vi "Add PV Protocols to FGV.vi"(8 "Error In":errorcluster, 10 "PV Protocol Section":string="PV_Protocols", 11 "CS++Factory":refnum<class "CS++Factory.lvclass">) -> (0 "Error Out":errorcluster)   [LabVIEW 2014, in "CS++ProcessVariables.lvlib"]
doc: "Read PV Protocols from configuration data to FGV."
uses:
  CS++ProcessVariables.lvlib
  CS++BaseClasses/Factory/CS++Factory.lvclass
  PVConnection/PVConnection.lvclass
  Libraries/Base/FGV Action.ctl
  Libraries/Base/CS++Base.lvlib
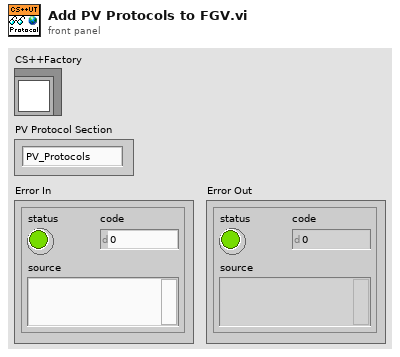
[diagram p1: front panel]
types:
  T1 = typedef "CS++Base.lvlib/FGV Action.ctl" = enum16{"add", "replace", "read", "remove", "reset", "get attributes"}
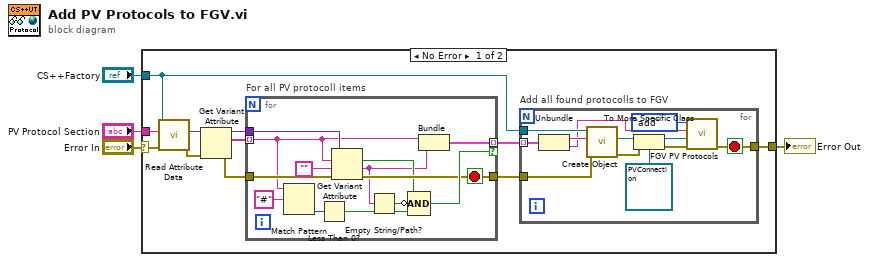
[diagram p0: block diagram]
diagram:
  n1 = case shown="No Error" "Error In" {
    selector: "Error In" -> [w5 w41]
    tunnel: "PV Protocol Section" -> [w8 _]
    tunnel: "CS++Factory" -> [w7 _]
    tunnel: [w6 w41] -> w2
    frame No Error {
      n2 = call-dynamic "Read Attribute Data.vi"("error in (no error)"=w5, "Object Name"=w8, "CS++Factory in"=w7) -> ("error out"=w15:errorcluster, "Attribute Data"=w14:variant)  [unwired: 6 in, 1 out]
      n3 = Get Variant Attribute(Variant=w14, error in=w15) -> (duplicate Variant=w12:variant, names=w13:string[], error out=w11:errorcluster)  [unwired: 2 in, 1 out]
      n4 = for "For all PV protocoll items" {
        tunnel: w13 -> [w36] mode=indexing
        tunnel: [w38] -> w9 mode=indexing if=w37
        tunnel: w12 -> [w40]
        tunnel: w11 -> [w39]
        tunnel: [w35] -> w10
        stop <- w35 stop-if-true
        n5 = Match Pattern(string=w36, regular expression="#") -> (offset past match=w33:i32)  [unwired: 1 in, 3 out]
        n6 = Less Than 0?(x=w33) -> (x < 0?=w32:bool)
        n7 = Get Variant Attribute(Variant=w40, name=w36, default value (empty Variant)="", error in=w39) -> (found=w30:bool, value=w28:string, error out=w35:errorcluster)  [unwired: 1 out]
        n8 = Empty String/Path?(string/path=w28) -> (empty?=w29:bool)
        n9 = Compound Arithmetic op=AND(w30, invert w29, w32) -> (w37:bool)
        n10 = Bundle(w36, w28) -> (w38:cluster{string, string})  [unwired: 1 in]
      }
      n11 = for "Add all found protocolls to FGV" {
        tunnel: w10 -> [w22]
        tunnel: w9 -> [w27] mode=indexing
        tunnel: w7 -> [w25]
        tunnel: [w17] -> w6
        stop <- w17 stop-if-true
        n12 = Unbundle(w27) -> (w26:string, w18:string)
        n13 = call "Create Object.vi"("error in (no error)"=w22, "Object Name"=w26, "CS++Factory in"=w25) -> ("error out"=w23:errorcluster, "LabVIEW Object"=w24:refnum<class>)  [unwired: 5 in, 2 out]
        n14 = To More Specific Class(target class=refnum<class "PVConnection.lvclass"> refnum ("CS++ProcessVariables.lvlib:PVConnection.lvclass"), reference=w24, error in=w23) -> (specific class reference=w19:refnum<class "PVConnection.lvclass">, error out=w20:errorcluster)
        n15 = call "FGV PV Protocols.vi"("Error In"=w20, "PVConnection in"=w19, "PV Protocol"=w18, "Action (read)"=FGV_Action."add") -> ("Error Out"=w17:errorcluster)  [unwired: 3 in, 4 out]
      }
    }
    frame Error {
    }
  }
  "Error Out" <- w2
